vi "CC Restore Previous Setup.vi"() -> (2 "Select File":path, 3 "Restored?":bool)   [LabVIEW 2024]
uses:
  <vilib>/Utility/miscctls.llb/LVRowAndColumnUnsignedTypeDef.ctl
  ccb2f664-5ae3-4a0e-bf14-ffdedb879ad2.vi
  <vilib>/Comparison/Less/Less Functor/Less Functor.lvclass
panel:
  in  "Cancel":bool
  out "Contents":string
  in  "Restore":bool
  in  "Previous Setups":i32(listbox)
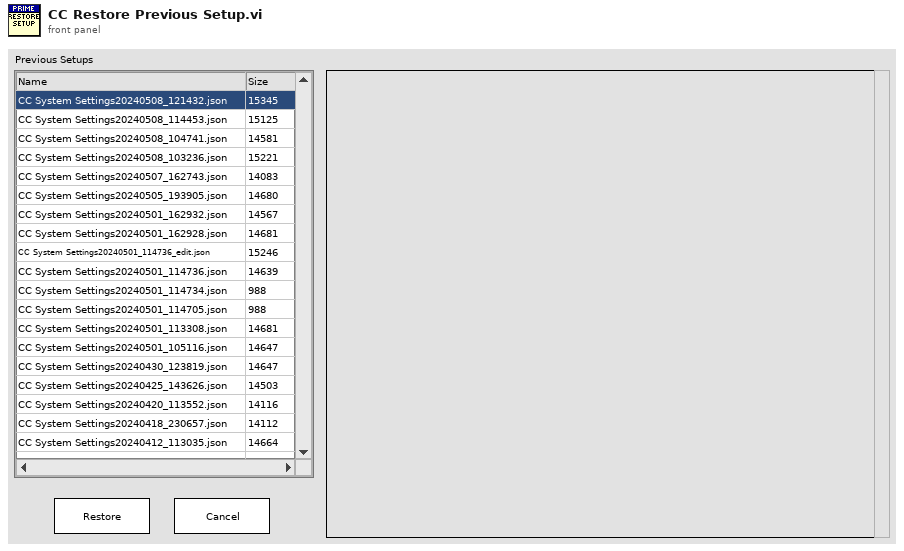
[diagram p1: front panel]
types:
  T1 = cluster{"state":refnum<user-event>, "Path":path, "Select File":path, "Restored?":bool}
  T2 = typedef "LVRowAndColumnUnsignedTypeDef.ctl" = cluster{"Row":u32, "Column":u32}
  T3 = enum32{"invalid app kind", "Development System", "Run Time System", "Student Edition", "Embedded LabVIEW", "Evaluation", "Custom"}
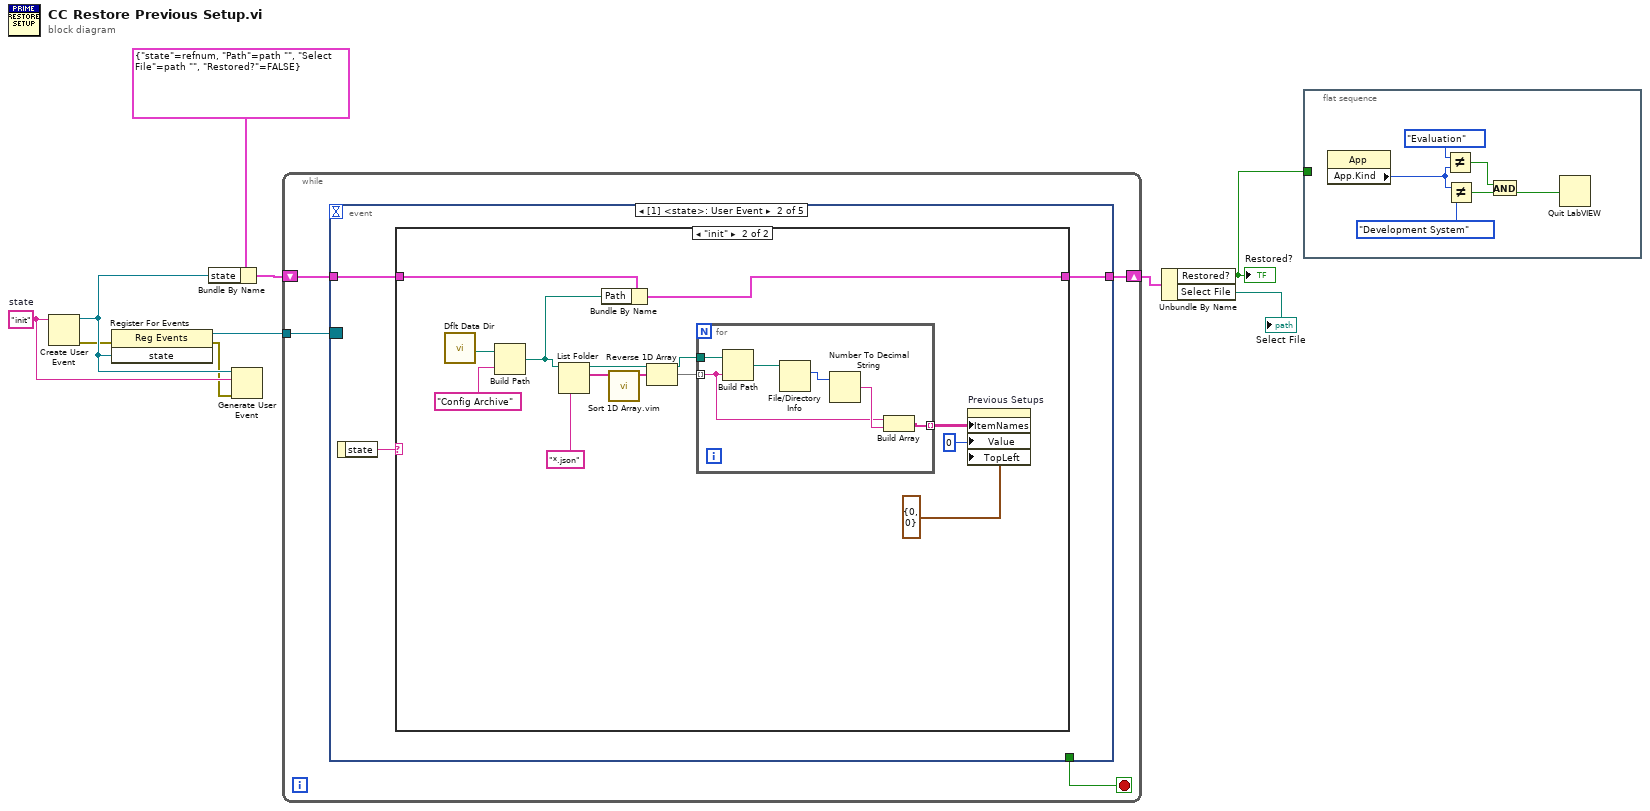
[diagram p0: block diagram]
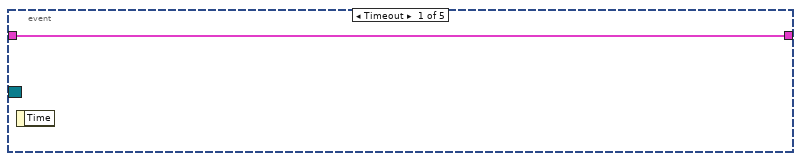
[diagram p2: hidden frame]
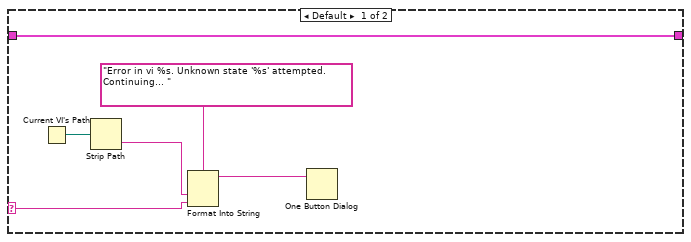
[diagram p3: hidden frame]
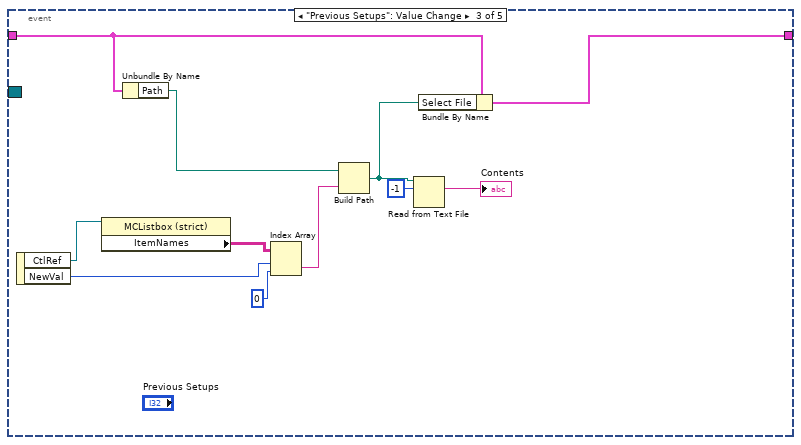
[diagram p4: hidden frame]
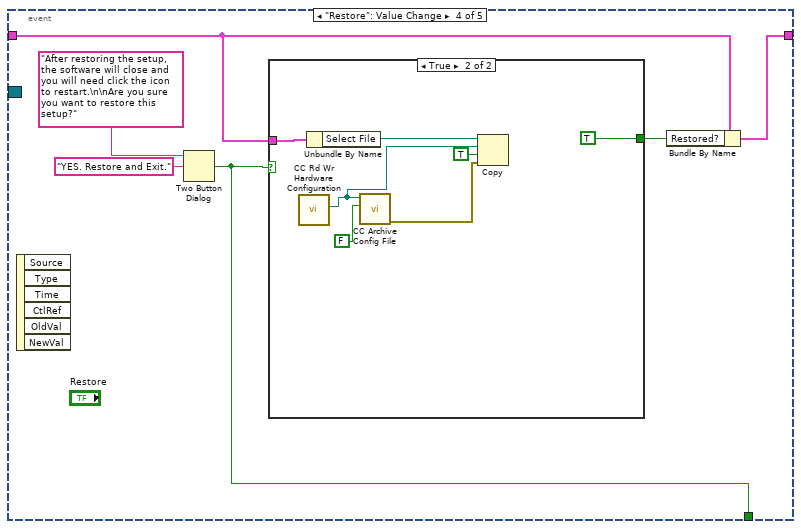
[diagram p5: hidden frame]
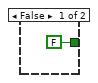
[diagram p6: hidden frame]
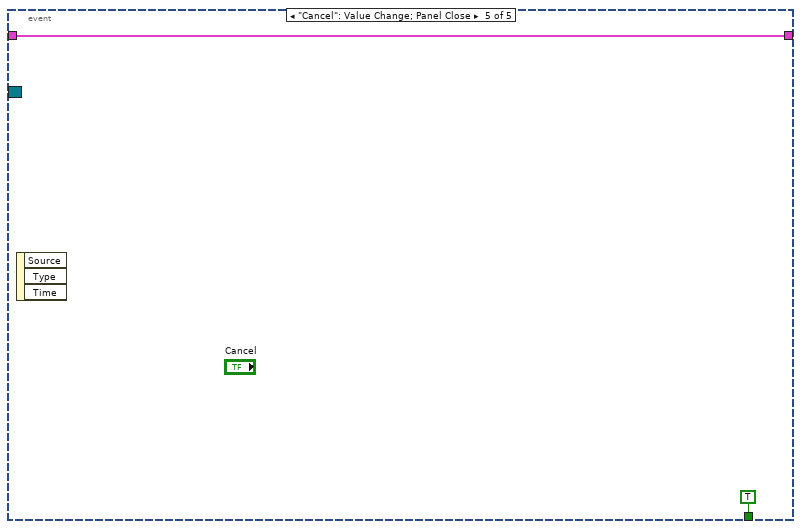
[diagram p7: hidden frame]
diagram:
  w6 = "init"  # state
  n1 = Create User Event(user event datatype=w6) -> (user event=w8:refnum<user-event>, error out=w4:errorcluster)  [unwired: 1 in]
  n2 = register-events(error in=w4, w8) -> (reference out=w7:refnum<event-registration>, error out=w5:errorcluster)  [unwired: 1 in]
  n3 = Bundle By Name(cluster=T1 {"state"=refnum, "Path"=path "", "Select File"=path "", "Restored?"=FALSE}, "state"=w8) -> (w9:T1)
  n4 = Generate User Event(user event=w8, event data cluster=w6, error in=w5) -> ()  [unwired: 1 in, 2 out]
  n5 = while {
    tunnel: w7 -> [w14]
    shift-right: [w12] -> w3
    shift-left: w9 -> [w13]
    stop <- w11 stop-if-true
    n6 = event shown="[1] <state>: User Event" {
      selector: w14 -> [_ _ _ _ _]
      dyn-events: _ -> [_ _ _ _ _]
      timeout: _ -> [_ _ _ _ _]
      tunnel: w13 -> [w15 w17 w44 w55 w70]
      tunnel: [w15 w16 w45 w56 w70] -> w12
      tunnel: [_ _ _ w58 TRUE ("Close")] -> w11
      event Timeout {
        n7 = event-data() -> ()  [unwired: 1 in, 1 out]
      }
      event User Event {
        n8 = event-data() -> ("state"=w18:string)  [unwired: 1 in]
        n9 = case shown="\"init\"" w18 {
          selector: w18 -> [w23 _]
          tunnel: w17 -> [w19 w30]
          tunnel: [w19 w31] -> w16
          frame Default {
            n10 = Current VI's Path() -> (path=w22:path)
            n11 = Strip Path(path=w22) -> (name=w21:string)  [unwired: 1 out]
            n12 = Format Into String(format string="Error in vi %s. Unknown state '%s' attempted. Continuing... ", w21, w23) -> (resulting string=w20:string)  [unwired: 2 in, 1 out]
            n13 = One Button Dialog(message=w20) -> ()  [unwired: 1 in, 1 out]
          }
          frame "init" {
            n14 = call <vilib>:"Dflt Data Dir.vi"() -> ("App:Default Data Directory"=w37:path)
            n15 = Build Path(base path=w37, name or relative path="Config Archive") -> (appended path=w32:path)
            n16 = List Folder(path=w32, pattern="*.json") -> (path out=w34:path, filenames=w29:string[])  [unwired: 2 in, 2 out]
            n17 = Bundle By Name(cluster=w30, "Path"=w32) -> (w31:T1)
            n18 = call "Sort 1D Array.vim"("unsorted array"=w29) -> ("sorted array"=w28:string[])  [unwired: 10 in]
            n19 = Reverse 1D Array(array=w28) -> (reversed array=w26:string[])
            n20 = for {
              tunnel: w26 -> [w39] mode=indexing
              tunnel: w34 -> [w43]
              tunnel: [w38] -> w33 mode=indexing
              n21 = Build Path(base path=w43, name or relative path=w39) -> (appended path=w42:path)
              n22 = File/Directory Info(path=w42) -> (size=w41:i64)  [unwired: 1 in, 6 out]
              n23 = Number To Decimal String(number=w41) -> (decimal integer string=w40:string)  [unwired: 1 in]
              n24 = Build Array(w39, w40) -> (w38:string[])
            }
            n25 = property on="Previous Setups" class="MCListbox (strict)"("ItemNames"=w33, "Value"=0 ("Previous Setups"), "TopLeft"=T2 {"Row"=0, "Column"=0} ("Top Left Visible Cell")) -> ()  [unwired: 2 in, 2 out]
          }
        }
      }
      event "Previous Setups": Value Change {
        n26 = event-data() -> ("CtlRef"=w54:refnum<vi>, "NewVal"=w52:i32)  [unwired: 1 in]
        n27 = property class="MCListbox (strict)"(reference=w54) -> ("ItemNames"=w53:string[][])  [unwired: 1 in, 2 out]
        n28 = Unbundle By Name(w44) -> ("Path"=w50:path)
        n29 = Index Array(array=w53, index (row)=w52, index (col)=0 ("disabled index (col)")) -> (element=w49:string)
        n30 = Build Path(base path=w50, name or relative path=w49) -> (appended path=w46:path)
        n31 = Read from Text File(file (use dialog)=w46, count=-1) -> (text=→"Contents":string)  [unwired: 2 in, 3 out]
        n32 = Bundle By Name(cluster=w44, "Select File"=w46) -> (w45:T1)
      }
      event "Restore": Value Change {
        n33 = event-data() -> ()  [unwired: 1 in, 6 out]
        n34 = Two Button Dialog(message="After restoring the setup, the software will close and you will need click the icon to restart.\n\nAre you sure you want to restore this setup?", 2:"YES. Restore and Exit." ("T button name (\"OK\")")) -> (T button?=w58:bool)  [unwired: 1 in]
        n35 = case shown="True" w58 {
          tunnel: w55 -> [_ w68]
          tunnel: [FALSE TRUE] -> w57
          frame False {
          }
          frame True {
            n36 = call "CC Rd Wr Hardware Configuration.vi"() -> ("File"=w65:path)  [unwired: 8 in, 3 out]
            n37 = Unbundle By Name(w68) -> ("Select File"=w66:path)
            n38 = call "CC Archive Config File.vi"("Move?"=FALSE, "config file"=w65) -> ("error out"=w63:errorcluster)  [unwired: 9 in]
            n39 = Copy(8:w63, 9:TRUE ("overwrite (F)"), 10:w65, 11:w66) -> ()  [unwired: 1 in, 3 out]
          }
        }
        n40 = Bundle By Name(cluster=w55, "Restored?"=w57) -> (w56:T1)
      }
      event "Cancel": Value Change; Panel Close {
        n41 = event-data() -> ()  [unwired: 1 in, 3 out]
      }
    }
  }
  n42 = Unbundle By Name(w3) -> ("Restored?"=w1:bool, "Select File"=→"Select File":path)
  "Restored?" <- w1
  n43 = flat-sequence {
    tunnel: w1 -> [_]
    frame #0 {
      n44 = property class="App"() -> ("App.Kind"=w71:T3)  [unwired: 2 in, 2 out]
      n45 = Not Equal?(x=T3."Evaluation" ("y"), y=w71) -> (x != y?=w72:bool)
      n46 = Not Equal?(x=w71, y=T3."Development System") -> (x != y?=w75:bool)
      n47 = And(x=w72, y=w75) -> (x .and. y?=w73:bool)
      n48 = Quit LabVIEW(quit? (T)=w73) -> ()
    }
  }
